vi "SetDIRDSC.vi"(8 "error in (no error)":errorcluster, 10 "dir":u8, 11 "DSCNumber":u8) -> (0 "error out":errorcluster)   [LabVIEW 2015, in "ESLSCDLL.lvlib"]
uses:
  ESLSCDLL.lvlib
  Globals.vi
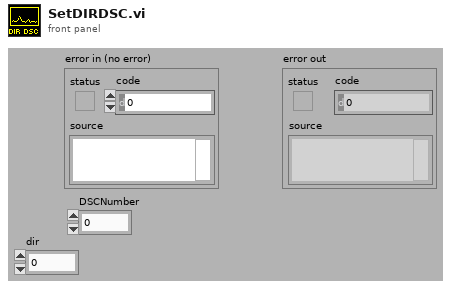
[diagram p1: front panel]
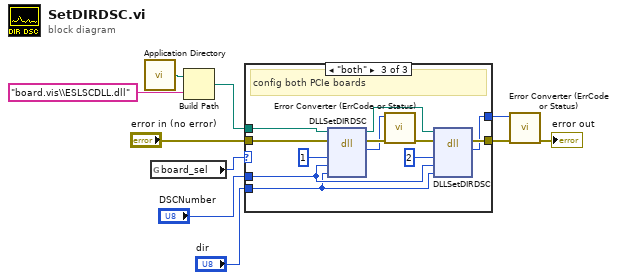
[diagram p0: block diagram]
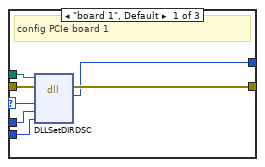
[diagram p2: hidden frame]
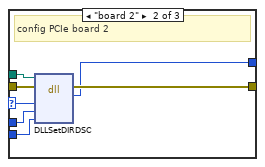
[diagram p3: hidden frame]
diagram:
  n1 = call <vilib>:"Application Directory.vi"() -> ("Application Directory"=w5:path)
  n2 = global read "Globals.vi" "board_sel"() -> (w6:enum32{"0", "board 1", "board 2", "both"})
  n3 = Build Path(base path=w5, name or relative path="board.vis\\ESLSCDLL.dll") -> (appended path=w3:path)
  n4 = case shown="\"both\"" w6 {
    selector: w6 -> [w17 w24 _]
    tunnel: "error in (no error)" -> [w16 w23 w34]
    tunnel: [w15 w22 w30] -> w8
    tunnel: [w14 w21 w29] -> w7
    tunnel: w3 -> [w13 w20 w28]
    tunnel: "DSCNumber" -> [w12 w19 w26]
    tunnel: "dir" -> [w11 w18 w25]
    frame "board 1", Default {
      # "config PCIe board 1"
      n5 = dll-call lib="C:/ENTW/PCIE/LV64/board.vis/ESLSCDLL.dll" fn="DLLSetDIRDSC" ("lwlscdll.dll:DLLWriteLongS0")(path in=w13, error in=w16, "drv"=w17, "DSCNumber"=w12, "dir"=w11) -> (error out=w15:errorcluster, "es_status_codes"=w14:i32)  [unwired: 4 in, 1 out]
    }
    frame "board 2" {
      # "config PCIe board 2"
      n6 = dll-call lib="C:/ENTW/PCIE/LV64/board.vis/ESLSCDLL.dll" fn="DLLSetDIRDSC" ("lwlscdll.dll:DLLWriteLongS0")(path in=w20, error in=w23, "drv"=w24, "DSCNumber"=w19, "dir"=w18) -> (error out=w22:errorcluster, "es_status_codes"=w21:i32)  [unwired: 4 in, 1 out]
    }
    frame "both" {
      # "config both PCIe boards"
      n7 = dll-call lib="C:/ENTW/PCIE/LV64/board.vis/ESLSCDLL.dll" fn="DLLSetDIRDSC" ("lwlscdll.dll:DLLWriteLongS0")(path in=w28, error in=w34, "drv"=u32 1, "DSCNumber"=w26, "dir"=w25) -> (path out=w27:path, error out=w33:errorcluster, "es_status_codes"=w32:i32)  [unwired: 4 in]
      n8 = call "Error Converter (ErrCode or Status).vi"("error in (no error)"=w33, "error code"=w32) -> ("error out"=w31:errorcluster)  [unwired: 9 in]
      n9 = dll-call lib="C:/ENTW/PCIE/LV64/board.vis/ESLSCDLL.dll" fn="DLLSetDIRDSC" ("lwlscdll.dll:DLLWriteLongS0")(path in=w27, error in=w31, "drv"=u32 2, "DSCNumber"=w26, "dir"=w25) -> (error out=w30:errorcluster, "es_status_codes"=w29:i32)  [unwired: 4 in, 1 out]
    }
  }
  n10 = call "Error Converter (ErrCode or Status).vi"("error in (no error)"=w8, "error code"=w7) -> ("error out"=→"error out":errorcluster)  [unwired: 9 in]
